vi "题目一.vi"() -> ()   [LabVIEW 2017]
panel:
  out "添加的数组":i32[](array[numeric])
  out "元素 4":i32
  out "元素 3":i32
  out "元素 2":i32
  out "元素":i32
  out "数组":dbl[](array[numeric])
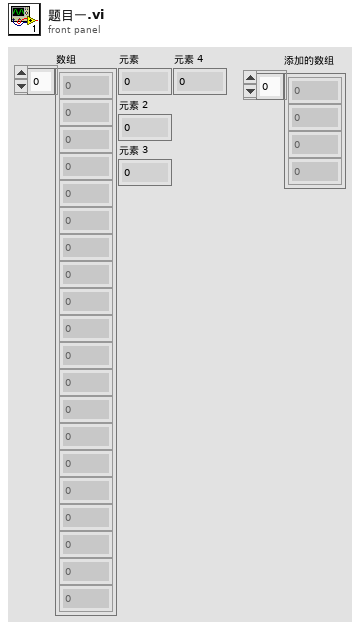
[diagram p1: front panel]
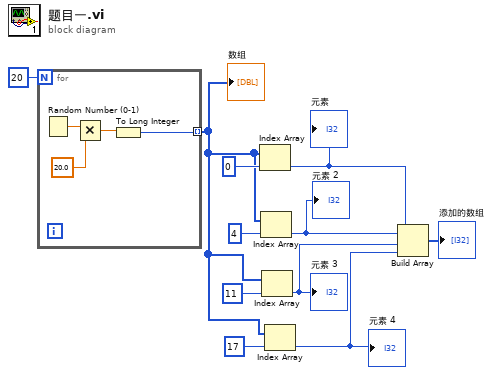
[diagram p0: block diagram]
diagram:
  n1 = for {
    N: 20 -> [_]
    tunnel: [w12] -> w6 mode=indexing
    n2 = Random Number (0-1)() -> (number: 0 to 1=w15:dbl)
    n3 = Multiply(x=w15, y=20.0) -> (x*y=w13:dbl)
    n4 = To Long Integer(number=w13) -> (32bit integer=w12:i32)
  }
  "数组" <- w6
  n5 = Index Array(array=w6, index=0 ("索引")) -> (element=w3:i32)
  "元素" <- w3
  n6 = Index Array(array=w6, index=4 ("索引")) -> (element=w4:i32)
  "元素 2" <- w4
  n7 = Index Array(array=w6, index=11 ("索引")) -> (element=w1:i32)
  "元素 3" <- w1
  n8 = Index Array(array=w6, index=17 ("索引")) -> (element=w5:i32)
  "元素 4" <- w5
  n9 = Build Array(w3, w4, w1, w5) -> (→"添加的数组":i32[])
